vi "RoundNum.vi"(1 "Decimal Places":i32, 2 "Unrounded Number":dbl format="%#_13g") -> (0 "Rounded Number":dbl format="%#_13g")   [LabVIEW 2017]
uses:
  <vilib>/express/express arith-compare/Formula/XNode/ExpressFormulaBlockNode.xnode
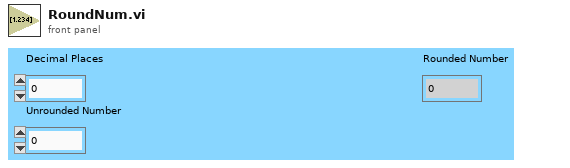
[diagram p1: front panel]
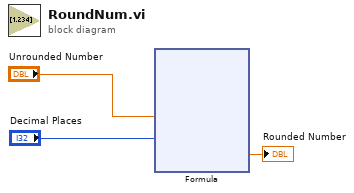
[diagram p0: block diagram]
diagram:
  n1 = xnode "Formula"("X"="Unrounded Number", "Y"="Decimal Places") -> ("Result"=→"Rounded Number":dbl)  [unwired: 1 in, 1 out]
